vi "Settings.vi"(8 "error in (no error)":errorcluster) -> (0 "error out":errorcluster)   [LabVIEW 2023]
uses:
  <vilib>/Utility/config.llb/Config Data RefNum.ctl
  CTLs/FGV Actions.ctl
  a5ac09e5-38d3-43bc-9feb-68748838b8f7.vi
  <vilib>/Utility/config.llb/Write Key (String).vi
  <vilib>/Utility/config.llb/Read Key (String).vi
  <vilib>/Utility/inputDevices.llb/closeKeyboard.vi
  <vilib>/Utility/inputDevices.llb/keyboardAcquire.vi
  FaKI State Machine/FaKI State Machine.lvlib
  <vilib>/Utility/config.llb/NI_LVConfig.lvlib
panel:
  in  "Reset":bool
  in  "Save":bool
  in  "Current Webhooks":string[][](table)
  in  "Start/Stop":bool
  in  "Exit":bool
  # "Change Hotkey\nPress \"Start Listening\" and hold down a key combination for five seconds to assign it as your new application Hotkey."
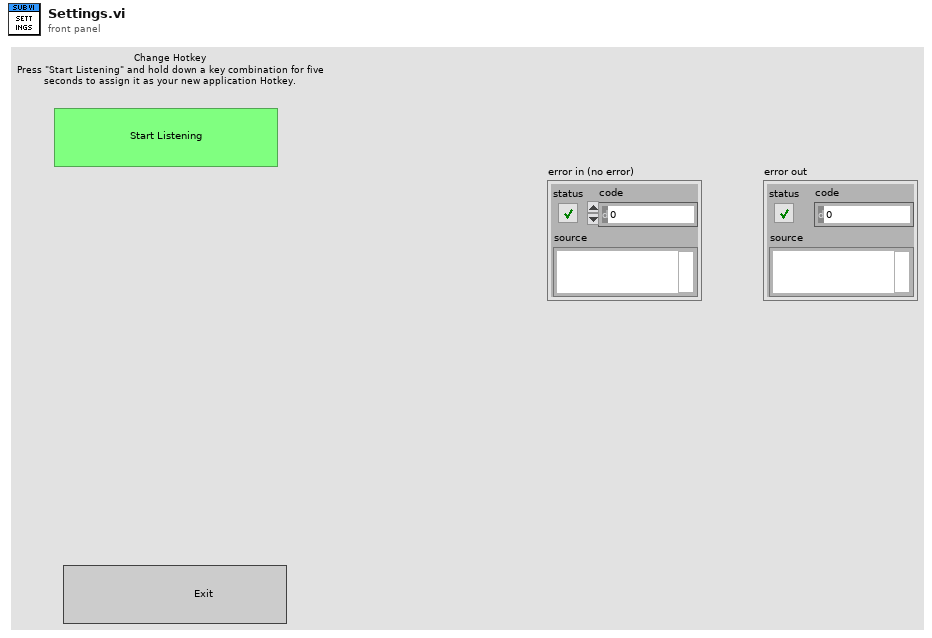
[diagram p1: front panel]
types:
  T1 = enum32{"Invalid", "Standard", "Closed", "Hidden", "Minimized", "Maximized"}
  T2 = enum32{"invalid app kind", "Development System", "Run Time System", "Student Edition", "Embedded LabVIEW", "Evaluation", "Custom"}
  T3 = typedef "FGV Actions.ctl" = enum16{"Read", "Write"}
  T4 = typedef "NI_LVConfig.lvlib/Config Data RefNum.ctl" = refnum<k1>
  T5 = cluster{"Core":cluster{"Current VI Reference":refnum<vi>, "Close Panel on Exit?":bool}, "Config":T4, "Keyboard":refnum<k1>, "Last":enum16{"0", "1", "2", "3", "4", "5", "6", "7", "8", "9", "A", "B", "C", "D", "E", "F", "G", "H", "I", "J", "K", "L", "M", "N", "O", "P", "Q", "R", "S", "T", "U", "V", "W", "X", "Y", "Z", "F1", "F2", "F3", "F4", "F5", "F6", "F7", "F8", "F9", "F10", "F11", "F12", "F13", "F14", "F15", "ADD", "BACK", "BACKSLASH", "CAPITAL", "COMMA", "DECIMAL", "DELETE", "DIVIDE", "DOWN", "END", "EQUALS", "ESCAPE", "GRAVE (`)", "HOME", "INSERT", "LBRACKET", "LCONTROL", "LEFT", "L ALT", "LSHIFT", "LWIN", "MINUS", "MULTIPLY", "NEXT", "NUMLOCK", "NUMPAD_0", "NUMPAD_1", "NUMPAD_2", "NUMPAD_3", "NUMPAD_4", "NUMPAD_5", "NUMPAD_6", "NUMPAD_7", "NUMPAD_8", "NUMPAD_9", "PAUSE", "PERIOD", "PRIOR (PG UP)", "RBRACKET", "RCONTROL", "RETURN", "RIGHT", "R ALT", "RSHIFT", "RWIN", "SCROLL", "SEMICOLON", "SLASH", "SPACE", "SUBTRACT", "TAB", "UP", "ENTER (num pad)", "' (quote)"}[]}
  T6 = enum16{"0", "1", "2", "3", "4", "5", "6", "7", "8", "9", "A", "B", "C", "D", "E", "F", "G", "H", "I", "J", "K", "L", "M", "N", "O", "P", "Q", "R", "S", "T", "U", "V", "W", "X", "Y", "Z", "F1", "F2", "F3", "F4", "F5", "F6", "F7", "F8", "F9", "F10", "F11", "F12", "F13", "F14", "F15", "ADD", "BACK", "BACKSLASH", "CAPITAL", "COMMA", "DECIMAL", "DELETE", "DIVIDE", "DOWN", "END", "EQUALS", "ESCAPE", "GRAVE (`)", "HOME", "INSERT", "LBRACKET", "LCONTROL", "LEFT", "L ALT", "LSHIFT", "LWIN", "MINUS", "MULTIPLY", "NEXT", "NUMLOCK", "NUMPAD_0", "NUMPAD_1", "NUMPAD_2", "NUMPAD_3", "NUMPAD_4", "NUMPAD_5", "NUMPAD_6", "NUMPAD_7", "NUMPAD_8", "NUMPAD_9", "PAUSE", "PERIOD", "PRIOR (PG UP)", "RBRACKET", "RCONTROL", "RETURN", "RIGHT", "R ALT", "RSHIFT", "RWIN", "SCROLL", "SEMICOLON", "SLASH", "SPACE", "SUBTRACT", "TAB", "UP", "ENTER (num pad)", "' (quote)"}[]
  T7 = cluster{"Current VI Reference":refnum<vi>, "Close Panel on Exit?":bool}
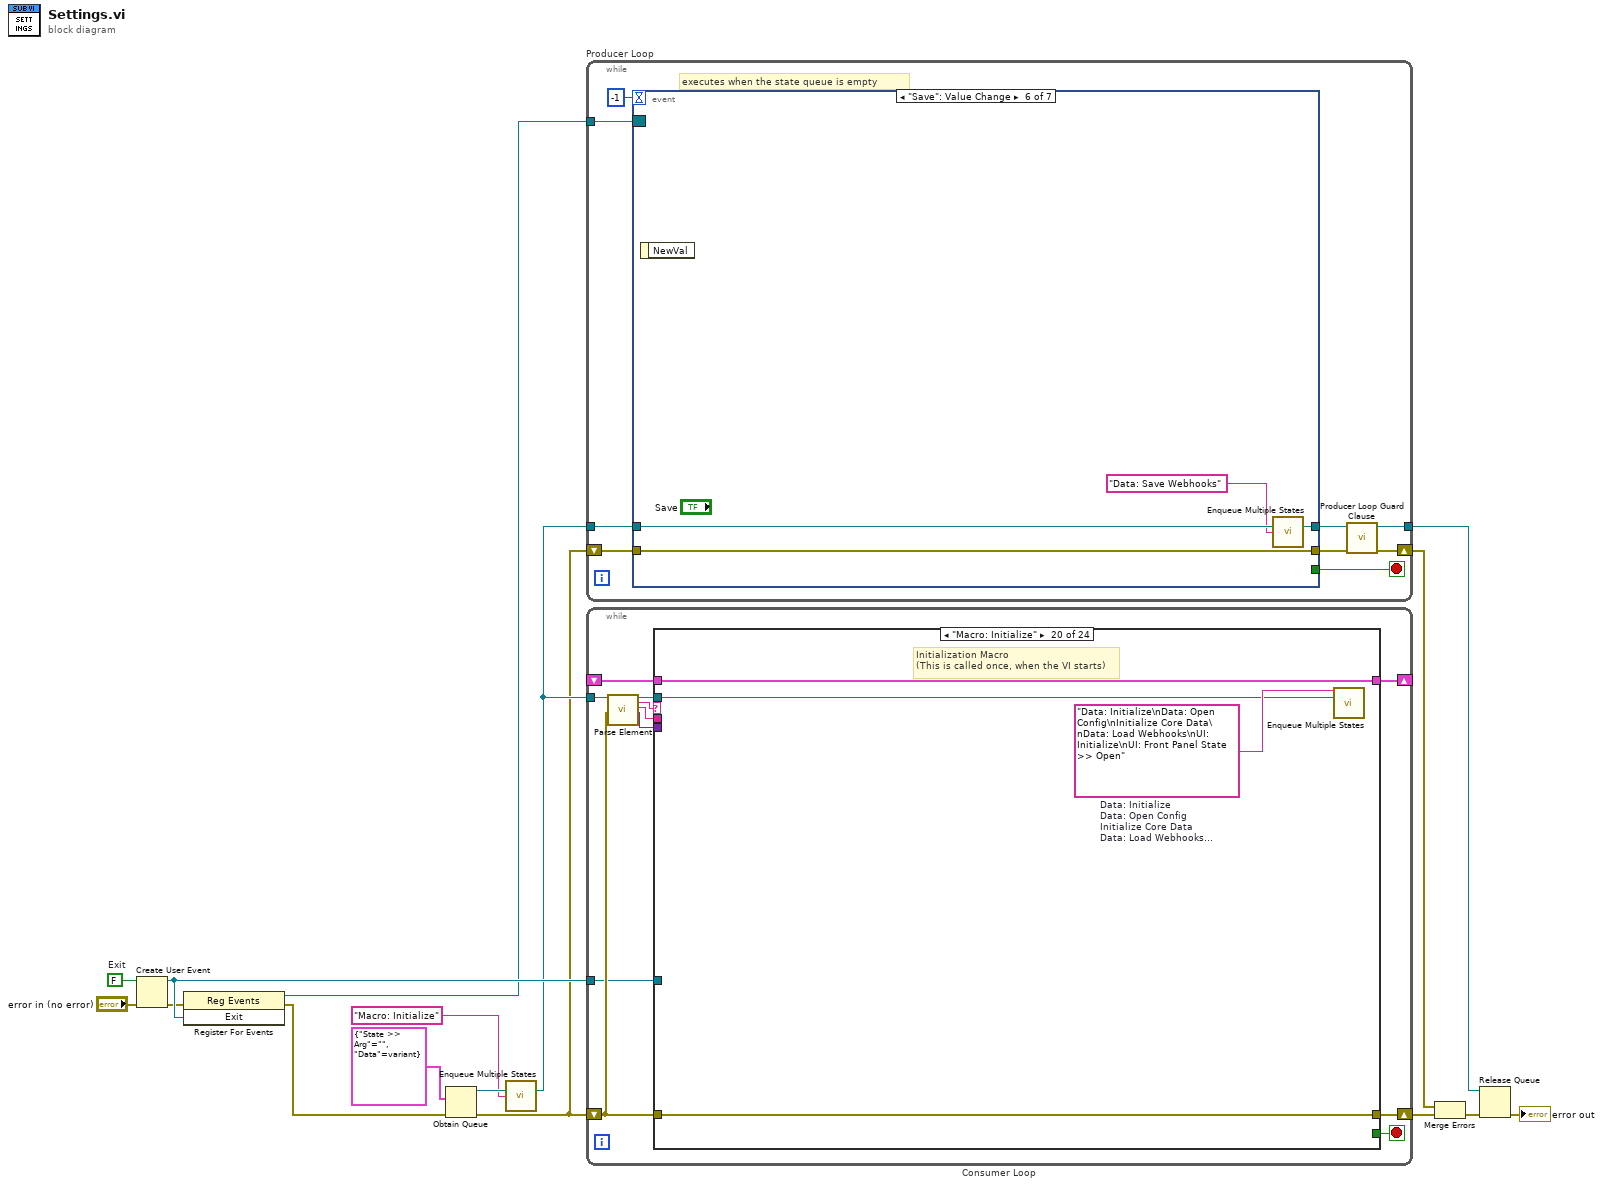
[diagram p0: block diagram]
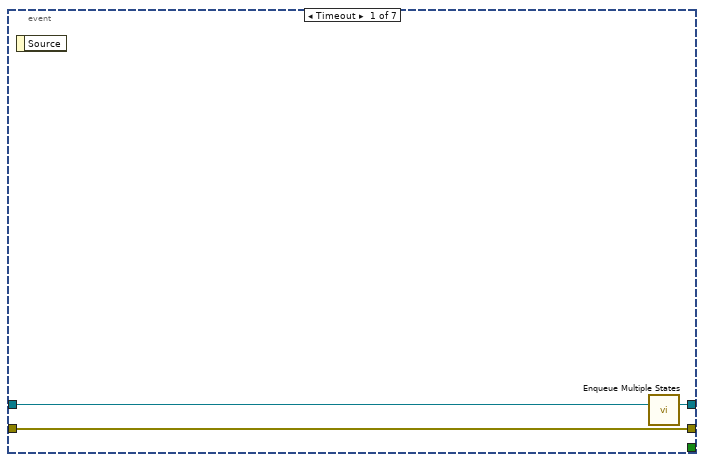
[diagram p2: hidden frame]
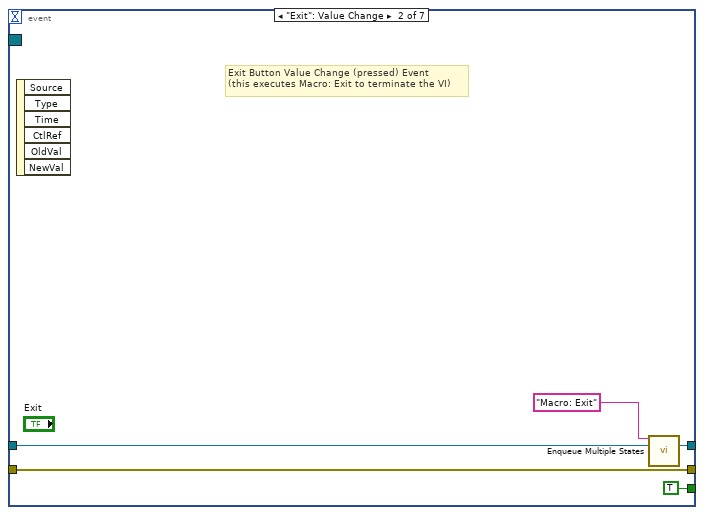
[diagram p3: hidden frame]
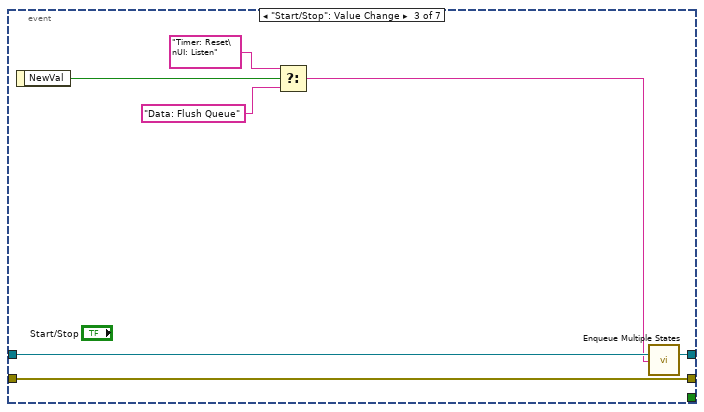
[diagram p4: hidden frame]
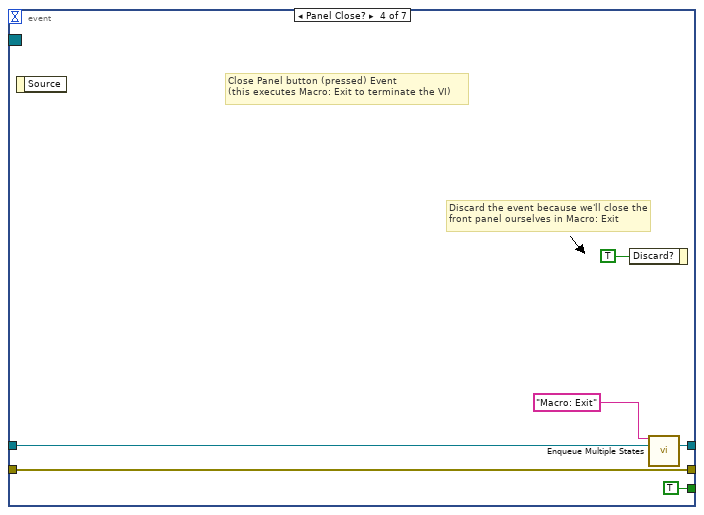
[diagram p5: hidden frame]
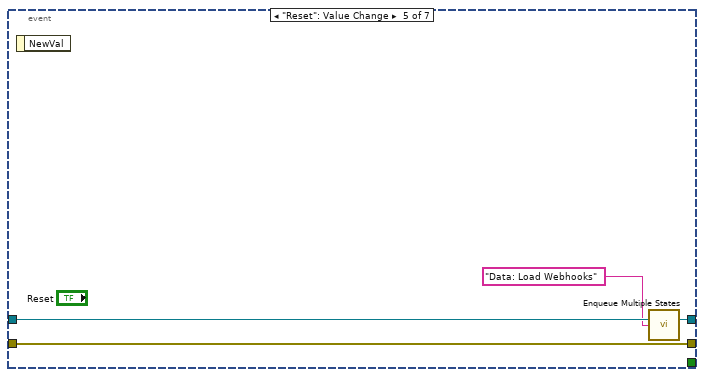
[diagram p6: hidden frame]
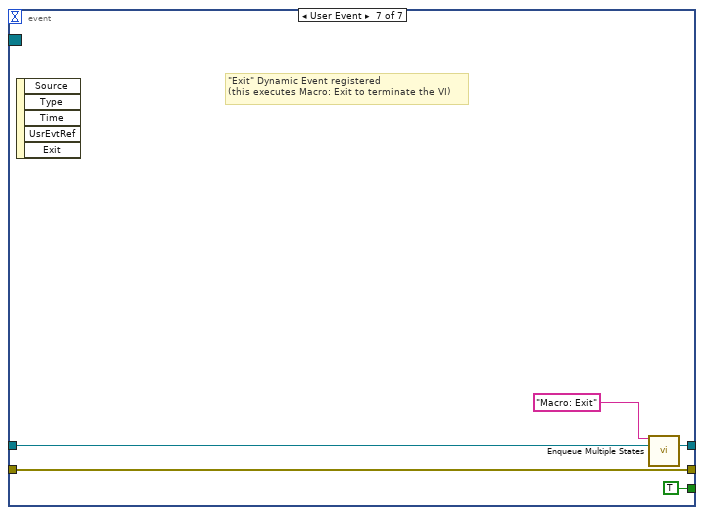
[diagram p7: hidden frame]
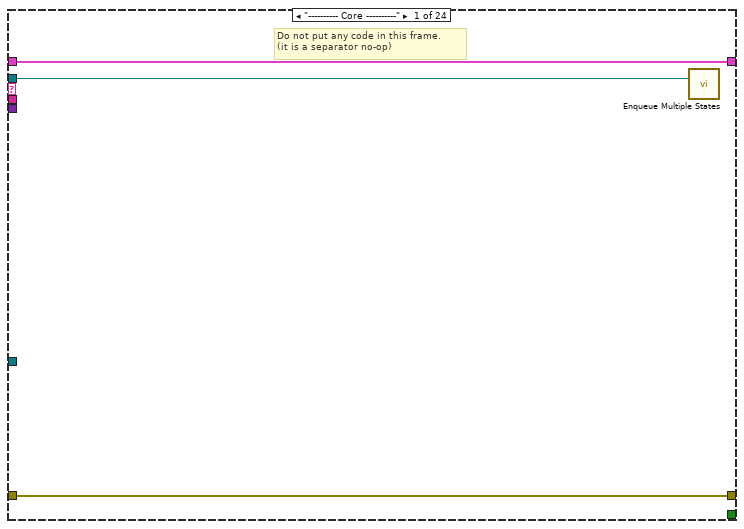
[diagram p8: hidden frame]
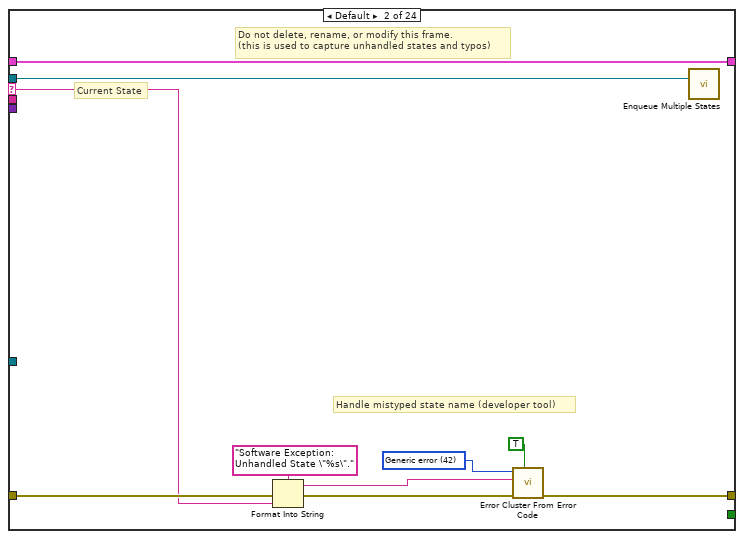
[diagram p9: hidden frame]
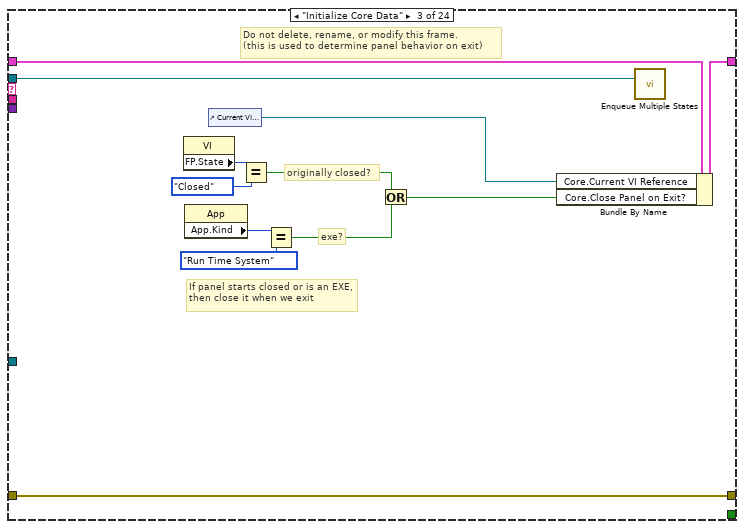
[diagram p10: hidden frame]
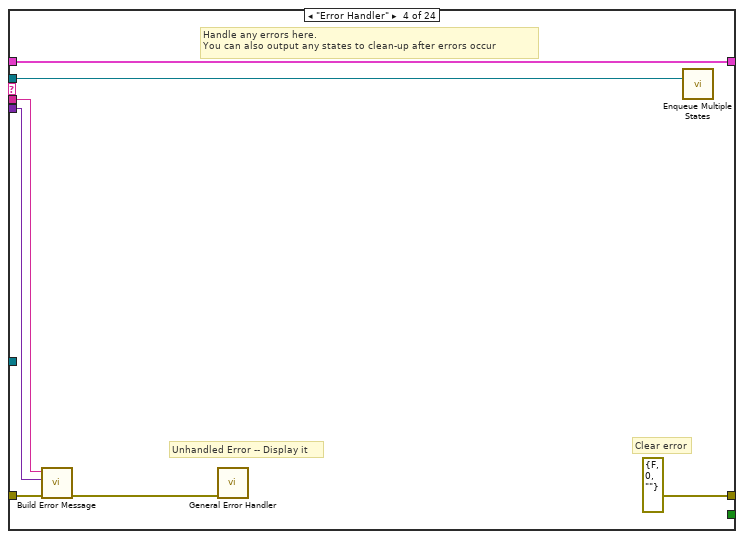
[diagram p11: hidden frame]
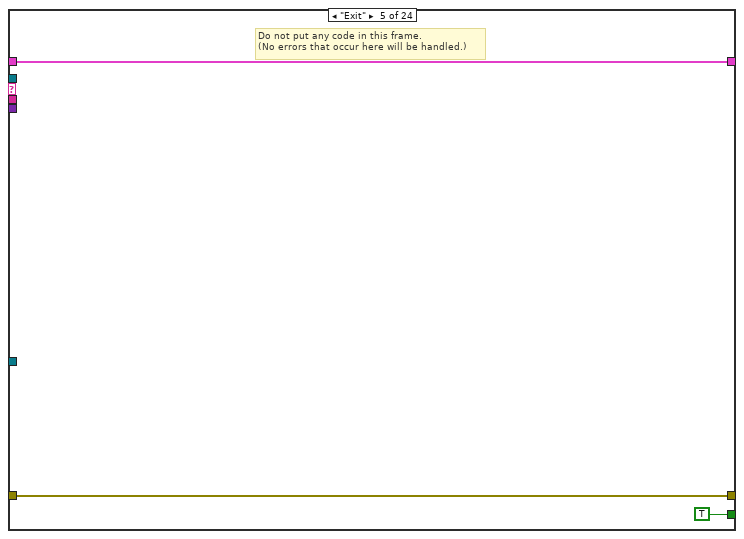
[diagram p12: hidden frame]
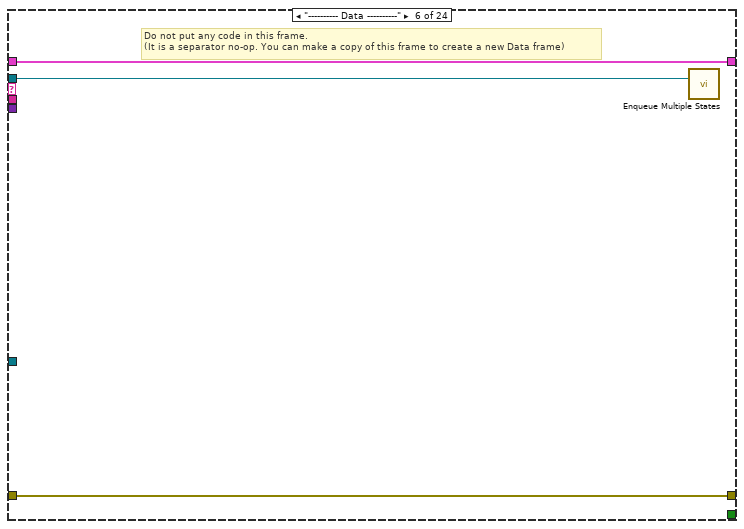
[diagram p13: hidden frame]
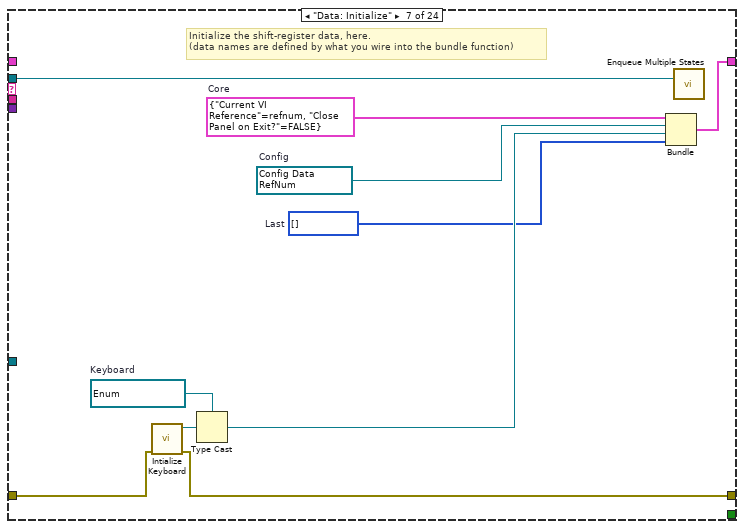
[diagram p14: hidden frame]
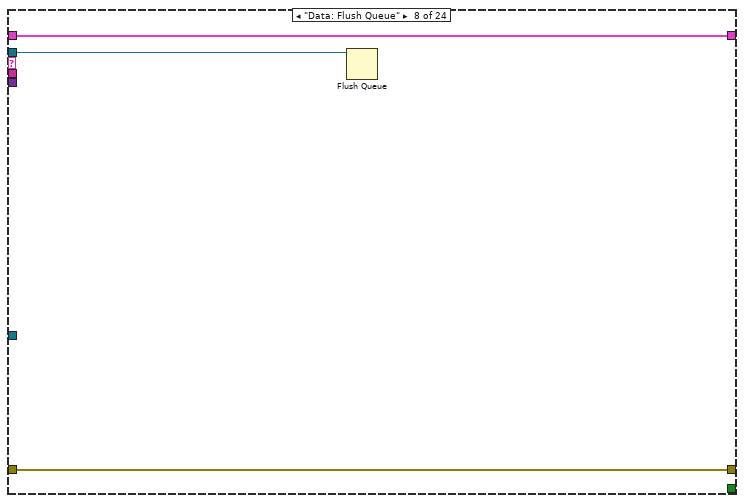
[diagram p15: hidden frame]
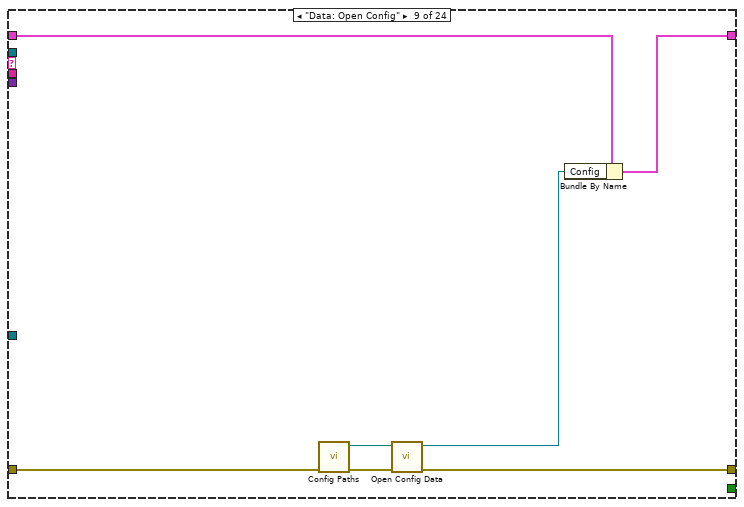
[diagram p16: hidden frame]
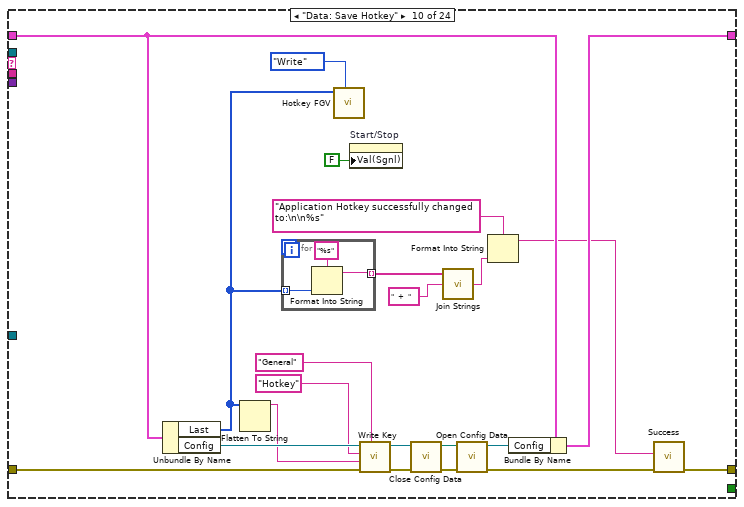
[diagram p17: hidden frame]
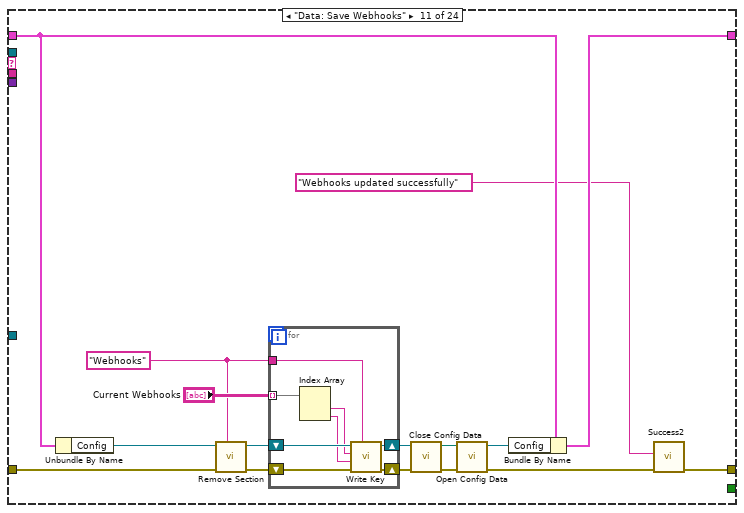
[diagram p18: hidden frame]
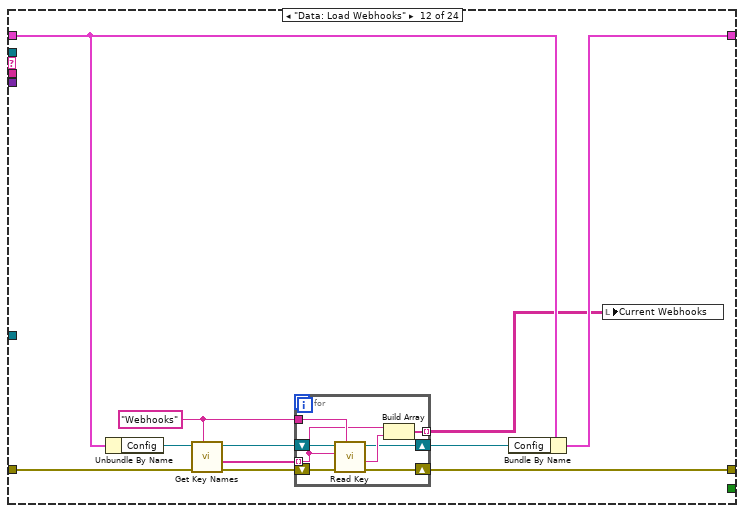
[diagram p19: hidden frame]
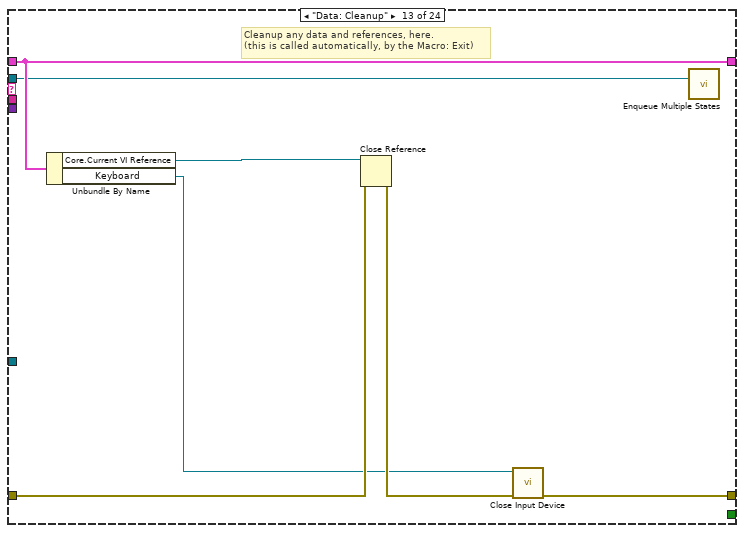
[diagram p20: hidden frame]
diagram:
  w13 = FALSE  # Exit
  n1 = Create User Event(user event datatype=w13, error in="error in (no error)") -> (user event=w16:refnum<user-event>, error out=w12:errorcluster)
  n2 = register-events(error in=w12, w16) -> (reference out=w15:refnum<event-registration>, error out=w14:errorcluster)  [unwired: 1 in]
  n3 = Obtain Queue(element data type=cluster{"State >> Arg":string, "Data":variant} {"State >> Arg"="", "Data"=variant}, error in (no error)=w14) -> (queue out=w6:refnum<queue>, error out=w3:errorcluster)  [unwired: 3 in, 1 out]
  n4 = call "Enqueue Multiple States.vi"("queue in"=w6, "State(s) at Back"="Macro: Initialize") -> ("queue out"=w7:refnum<queue>)  [unwired: 13 in]
  n5 = while "Producer Loop" {
    shift-right: [w20] -> w9
    shift-left: w3 -> [w25]
    tunnel: w15 -> [w17]
    tunnel: w7 -> [w23]
    tunnel: [w18] -> w11
    stop <- w22 stop-if-true
    # "executes when the state queue is empty"
    n6 = event shown="[5] \"Save\": Value Change" {
      selector: w17 -> [_ _ _ _ _ _ _]
      dyn-events: _ -> [_ _ _ _ _ _ _]
      timeout: -1 ("Timeout") -> [_ _ _ _ _ _ _]
      tunnel: [w26 w33 w40 w46 w50 w54 w59] -> w21
      tunnel: w25 -> [w26 w33 w40 w46 w50 w54 w59]
      tunnel: w23 -> [w27 w32 w39 w43 w49 w53 w57]
      tunnel: [w28 w30 w38 w42 w48 w52 w56] -> w19
      tunnel: [_ TRUE _ TRUE _ _ TRUE] -> w22
      event Timeout {
        n7 = event-data() -> ()  [unwired: 1 in, 1 out]
        n8 = call "Enqueue Multiple States.vi"("queue in"=w27) -> ("queue out"=w28:refnum<queue>)  [unwired: 14 in]
      }
      event "Exit": Value Change {
        # "Exit Button Value Change (pressed) Event\n(this executes Macro: Exit to terminate the VI)"
        n9 = event-data() -> ()  [unwired: 1 in, 6 out]
        n10 = call "Enqueue Multiple States.vi"("State(s) at Front"="Macro: Exit", "queue in"=w32) -> ("queue out"=w30:refnum<queue>)  [unwired: 13 in]
      }
      event "Start/Stop": Value Change {
        n11 = event-data() -> ("NewVal"=w37:bool)  [unwired: 1 in]
        n12 = Select(t="Timer: Reset\nUI: Listen", s=w37, f="Data: Flush Queue") -> (s? t:f=w34:string)
        n13 = call "Enqueue Multiple States.vi"("queue in"=w39, "State(s) at Back"=w34) -> ("queue out"=w38:refnum<queue>)  [unwired: 13 in]
      }
      event Panel Close? {
        # "Discard the event because we'll close the front panel ourselves in Macro: Exit"
        # "Close Panel button (pressed) Event\n(this executes Macro: Exit to terminate the VI)"
        n14 = event-data() -> ()  [unwired: 1 in, 1 out]
        n15 = event-data("Discard?"=TRUE) -> ()  [unwired: 1 in, 1 out]
        n16 = call "Enqueue Multiple States.vi"("State(s) at Front"="Macro: Exit", "queue in"=w43) -> ("queue out"=w42:refnum<queue>)  [unwired: 13 in]
      }
      event "Reset": Value Change {
        n17 = event-data() -> ()  [unwired: 1 in, 1 out]
        n18 = call "Enqueue Multiple States.vi"("queue in"=w49, "State(s) at Back"="Data: Load Webhooks") -> ("queue out"=w48:refnum<queue>)  [unwired: 13 in]
      }
      event "Save": Value Change {
        n19 = event-data() -> ()  [unwired: 1 in, 1 out]
        n20 = call "Enqueue Multiple States.vi"("queue in"=w53, "State(s) at Back"="Data: Save Webhooks") -> ("queue out"=w52:refnum<queue>)  [unwired: 13 in]
      }
      event User Event {
        # "\"Exit\" Dynamic Event registered\n(this executes Macro: Exit to terminate the VI)"
        n21 = event-data() -> ()  [unwired: 1 in, 5 out]
        n22 = call "Enqueue Multiple States.vi"("State(s) at Front"="Macro: Exit", "queue in"=w57) -> ("queue out"=w56:refnum<queue>)  [unwired: 13 in]
      }
    }
    n23 = call "Producer Loop Guard Clause.vi"("error in (no error)"=w21, "queue in"=w19) -> ("error out"=w20:errorcluster, "queue out"=w18:refnum<queue>)  [unwired: 8 in]
  }
  n24 = while "Consumer Loop" {
    shift-right: [w67] -> _
    shift-left: _ -> [w66]
    shift-right: [w70] -> w8
    shift-left: w3 -> [w69]
    tunnel: w7 -> [w65]
    tunnel: w16 -> [w60]
    stop <- w68 stop-if-true
    n25 = call "Parse Element.vi"("queue in"=w65, "error in (no error)"=w69) -> ("queue out"=w64:refnum<queue>, "State"=w63:string, "Arg"=w62:string, "Data"=w61:variant)  [unwired: 14 in]
    n26 = case shown="\"Macro: Initialize\"" w63 {
      selector: w63 -> [_ w75 _ _ _ _ _ _ _ _ _ _ _ _ _ _ _ _ _ _ _ _ _ _]
      tunnel: w64 -> [w71 w74 w84 w100 _ w106 w116 w121 _ _ _ _ w200 w204 w207 w210 w219 w294 w308 w311 w318 w324 _ w333]
      tunnel: w62 -> [_ _ _ w96 _ _ _ _ _ _ _ _ _ _ _ w211 w220 _ _ _ _ _ _ _]
      tunnel: w66 -> [w72 w77 w90 w101 w104 w107 _ w120 w125 w149 w168 w187 w201 w205 w208 w212 w222 w293 w309 w313 w322 w325 w331 w340]
      tunnel: [w73 w82 w95 errorcluster {"status"=FALSE, "code"=0, "source"=""} ("error out") w105 w108 w110 w119 w126 w132 w161 w180 w198 w206 w209 w213 w223 w302 w310 w314 w323 w326 w329 w338] -> w70
      tunnel: w69 -> [w73 w81 w95 w99 w105 w108 w113 w119 w127 w148 w158 w186 w203 w206 w209 w214 w224 w303 w310 w314 w323 w326 w330 w339]
      tunnel: [_ _ _ _ TRUE _ _ _ _ _ _ _ _ _ _ _ _ _ _ _ _ _ _ _] -> w68
      tunnel: [w72 w77 w94 w101 w104 w107 w118 w120 w124 w150 w169 w188 w201 w205 w208 w212 w222 w292 w309 w313 w322 w325 w331 w340] -> w67
      tunnel: w61 -> [_ _ _ w97 _ _ _ _ _ _ _ _ _ _ _ _ _ _ _ _ _ _ _ _]
      tunnel: w60 -> [_ _ _ _ _ _ _ _ _ _ _ _ _ _ _ _ _ _ _ _ _ _ _ _]
      frame "---------- Core ----------" {
        # "Do not put any code in this frame.\n(it is a separator no-op)"
        n27 = call "Enqueue Multiple States.vi"("queue in"=w71) -> ()  [unwired: 14 in, 1 out]
      }
      frame Default {
        w79 = 42 items=["No error", "Argument error", "Memory is full", "Out of zone", "End of file", "File already open", "Generic file I/O error", "File not found", "File permission error", "Disk is full", "Duplicate path", "Too many files open", "System feature not enabled", "Resource file not found", "Cannot add resource", "Resource not found", "Image not found", "Image memory error", "Pen does not exist", "Config type invalid", "Config token not found", "Config parse error", "Config memory error", "Bad external code format", "Bad external code offset", "External code not present", "Null window", "Destroy window error", "Null menu", "Print aborted", "Bad print record", "Print driver error", "Windows error during printing", "Memory error during printing", "Print dialog error", "Generic print error", "Invalid device refnum", "Device not found", "Device parameter error", "Device unit error", "Cannot open device", "Device call aborted", "Generic error", "Cancelled by user", "Object ID too low", "Object ID too high", "Object not in heap", "Unknown heap", "Unknown object (invalid DefProc)", "Unknown object (DefProc not in table)", "Message out of range", "Invalid (null) method", "Unknown message", "Manager call not supported", "Bad address", "Network operation in progress", "Network operation timed out", "Connection is busy", "Network attribute not supported", "Network error", "Address in use", "System out of memory", "Connection aborted", "Connection refused", "Not connected", "Already connected", "Connection closed", "Initialization error (interapplication manager)", "Bad occurrence", "Wait on unbound occurrence handler", "Occurrence queue overflow", "Datalog type conflict", "Unused", "Unrecognized type (interapplication manager)", "Memory corrupt", "Failed to make temporary DLL", "Old CIN version", "Drag socket not found", "Failed to load drop-object", "Failed to register OLE object", "Failed to release OLE object", "Format specifier type mismatch", "Unknown format specifier", "Too few format specifiers", "Too many format specifiers", "Scan failed", "Newer CIN version", "Error converting to variant", "Runtime menu error", "Password tampered", "Variant attribute not found", "Incompatible variant data type", "Event data is not available", "Event Store is not present", "Occurrence is not found", "Event Queue is not created", "Event info is not available", "Refnum passed is NULL", "Error retrieving Class GUID", "Error retrieving CoClass GUID", "Error retrieving TypeLib GUID.", "Bad built application magic bytes.", "Specific driver is different from the specific driver associated with the Logical Name.", "There is no session opened to the class driver.", "Max Error", "MAX - Error with config objects", "MAX - Error loading configuration", "MAX - Group not supported"]
        # "Current State"
        # "Do not delete, rename, or modify this frame.\n(this is used to capture unhandled states and typos)"
        # "Handle mistyped state name (developer tool)"
        n28 = Format Into String(format string="Software Exception: Unhandled State \"%s\"." ("message"), error in=w81, w75) -> (resulting string=w78:string, error out=w83:errorcluster)  [unwired: 1 in]
        n29 = call <vilib>:"Error Cluster From Error Code.vi"("show call chain? (False)"=TRUE, "error in (no error)"=w83, "error message (\"\")"=w78, "error code (0)"=w79) -> ("error out"=w82:errorcluster)  [unwired: 5 in]
        n30 = call "Enqueue Multiple States.vi"("queue in"=w74) -> ()  [unwired: 14 in, 1 out]
      }
      frame "Initialize Core Data" {
        # "Do not delete, rename, or modify this frame.\n(this is used to determine panel behavior on exit)"
        # "originally closed?"
        # "exe?"
        # "If panel starts closed or is an EXE, then close it when we exit"
        n31 = property class="VI"() -> ("FP.State"=w87:T1)  [unwired: 2 in, 2 out]
        n32 = property class="App"() -> ("App.Kind"=w93:T2)  [unwired: 2 in, 2 out]
        n33 = control-ref of="Current VI Reference"() -> (w88:refnum<vi>)
        n34 = Equal?(x=w87, y=T1."Closed" ("Front Panel Window:State")) -> (x = y?=w85:bool)
        n35 = Equal?(x=w93, y=T2."Run Time System" ("Application:Kind")) -> (x = y?=w91:bool)
        n36 = Or(x=w85, y=w91) -> (x .or. y?=w89:bool)
        n37 = Bundle By Name(cluster=w90, "Core.Current VI Reference"=w88, "Core.Close Panel on Exit?"=w89) -> (w94:T5)
        n38 = call "Enqueue Multiple States.vi"("queue in"=w84) -> ()  [unwired: 14 in, 1 out]
      }
      frame "Error Handler" {
        # "Unhandled Error -- Display it"
        # "Handle any errors here.\nYou can also output any states to clean-up after errors occur"
        # "Clear error"
        n39 = call "Build Error Message.vi"("error in (no error)"=w99, "Data"=w97, "Arg"=w96) -> ("error out"=w98:errorcluster)  [unwired: 8 in]
        n40 = call <vilib>:"General Error Handler.vi"("error in (no error)"=w98) -> ()  [unwired: 10 in, 5 out]
        n41 = call "Enqueue Multiple States.vi"("queue in"=w100) -> ()  [unwired: 14 in, 1 out]
      }
      frame "Exit" {
        # "Do not put any code in this frame.\n(No errors that occur here will be handled.)"
      }
      frame "---------- Data ----------" {
        # "Do not put any code in this frame.\n(It is a separator no-op. You can make a copy of this frame to create a new Data frame)"
        n42 = call "Enqueue Multiple States.vi"("queue in"=w106) -> ()  [unwired: 14 in, 1 out]
      }
      frame "Data: Initialize" {
        w109 = T6 [] items=["0", "1", "2", "3", "4", "5", "6", "7", "8", "9", "A", "B", "C", "D", "E", "F", "G", "H", "I", "J", "K", "L", "M", "N", "O", "P", "Q", "R", "S", "T", "U", "V", "W", "X", "Y", "Z", "F1", "F2", "F3", "F4", "F5", "F6", "F7", "F8", "F9", "F10", "F11", "F12", "F13", "F14", "F15", "ADD", "BACK", "BACKSLASH", "CAPITAL", "COMMA", "DECIMAL", "DELETE", "DIVIDE", "DOWN", "END", "EQUALS", "ESCAPE", "GRAVE (`)", "HOME", "INSERT", "LBRACKET", "LCONTROL", "LEFT", "L ALT", "LSHIFT", "LWIN", "MINUS", "MULTIPLY", "NEXT", "NUMLOCK", "NUMPAD_0", "NUMPAD_1", "NUMPAD_2", "NUMPAD_3", "NUMPAD_4", "NUMPAD_5", "NUMPAD_6", "NUMPAD_7", "NUMPAD_8", "NUMPAD_9", "PAUSE", "PERIOD", "PRIOR (PG UP)", "RBRACKET", "RCONTROL", "RETURN", "RIGHT", "R ALT", "RSHIFT", "RWIN", "SCROLL", "SEMICOLON", "SLASH", "SPACE", "SUBTRACT", "TAB", "UP", "ENTER (num pad)", "' (quote)"]  # Last
        w112 = T4 refnum items=["config data"]  # Config
        w114 = refnum<k1> refnum items=["KEYBOARD"]  # Keyboard
        w117 = T7 {"Current VI Reference"=refnum, "Close Panel on Exit?"=FALSE}  # Core
        # "Initialize the shift-register data, here.\n(data names are defined by what you wire into the bundle function)"
        n43 = call <vilib>:"Intialize Keyboard.vi"("error in (no error)"=w113) -> ("error out"=w110:errorcluster, "device ID"=w115:refnum<k1>)  [unwired: 9 in]
        n44 = Type Cast(type=w114, x=w115) -> (*(type *) &x=w111:refnum<k1>)
        n45 = Bundle("Core"=w117, "Config"=w112, "Keyboard"=w111, "Last"=w109) -> (w118:T5)  [unwired: 1 in]
        n46 = call "Enqueue Multiple States.vi"("queue in"=w116) -> ()  [unwired: 14 in, 1 out]
      }
      frame "Data: Flush Queue" {
        n47 = Flush Queue(queue=w121) -> ()  [unwired: 1 in, 3 out]
      }
      frame "Data: Open Config" {
        n48 = call "Config Paths.vi"("error in (no error)"=w127) -> ("error out"=w128:errorcluster, "Global Config"=w122:path)  [unwired: 7 in, 2 out]
        n49 = call <vilib>:"Open Config Data.vi"("error in (no error)"=w128, "configuration file path"=w122) -> ("error out"=w126:errorcluster, "refnum"=w123:T4)  [unwired: 7 in, 1 out]
        n50 = Bundle By Name(cluster=w125, "Config"=w123) -> (w124:T5)
      }
      frame "Data: Save Hotkey" {
        n51 = Unbundle By Name(w149) -> ("Last"=w130:T6, "Config"=w143:T4)
        n52 = Flatten To String(anything=w130) -> (data string=w142:string)  [unwired: 3 in, 2 out]
        n53 = for {
          tunnel: w130 -> [w152] mode=indexing
          tunnel: [w151] -> w138 mode=indexing
          n54 = Format Into String(format string="%s", w152) -> (resulting string=w151:string)  [unwired: 2 in, 1 out]
        }
        n55 = call "Hotkey FGV.vi"("Mode"=FGV_Actions."Write", "Hotkey"=w130) -> ()  [unwired: 7 in, 3 out]
        n56 = property on="Start/Stop" class="Bool (strict)"("Val(Sgnl)"=FALSE ("Value (Signaling)")) -> ()  [unwired: 2 in, 2 out]
        n57 = call-poly <vilib>:"Write Key.vi"("section"="General", "error in (no error)"=w148, "value"=w142, "key"="Hotkey", "refnum"=w143) -> ("error out"=w147:errorcluster, "refnum out"=w146:T4)  [unwired: 4 in, 1 out]
        n58 = call <vilib>:"Close Config Data.vi"("error in (no error)"=w147, "refnum"=w146) -> ("error out"=w144:errorcluster, "file path"=w145:path)  [unwired: 8 in]
        n59 = call <vilib>:"Join Strings.vi"("Separator (,)"="  +  ", "Strings In"=w138) -> ("String"=w135:string)  [unwired: 1 in]
        n60 = call <vilib>:"Open Config Data.vi"("error in (no error)"=w144, "configuration file path"=w145) -> ("error out"=w133:errorcluster, "refnum"=w139:T4)  [unwired: 7 in, 1 out]
        n61 = Format Into String(format string="Application Hotkey successfully changed to:\n\n%s", w135) -> (resulting string=w134:string)  [unwired: 2 in, 1 out]
        n62 = Bundle By Name(cluster=w149, "Config"=w139) -> (w150:T5)
        n63 = call "Success"("error in (no error)"=w133, "Message"=w134) -> ("error out"=w132:errorcluster)  [unwired: 8 in, 1 out]
      }
      frame "Data: Save Webhooks" {
        w155 = "Webhooks" ("section")
        n64 = Unbundle By Name(w168) -> ("Config"=w156:T4)
        n65 = call <vilib>:"Remove Section.vi"("section"=w155, "error in (no error)"=w158, "refnum"=w156) -> ("error out"=w154:errorcluster, "refnum out"=w157:T4)  [unwired: 6 in, 1 out]
        n66 = for {
          tunnel: w155 -> [w173]
          shift-right: [w176] -> w167
          shift-left: w154 -> [w177]
          tunnel: "Current Webhooks" -> [w172] mode=indexing
          shift-right: [w175] -> w166
          shift-left: w157 -> [w174]
          n67 = Index Array(array=w172) -> (element #1=w170:string, element #2=w171:string)  [unwired: 2 in]
          n68 = call-poly <vilib>:"Write Key.vi"("section"=w173, "error in (no error)"=w177, "value"=w171, "key"=w170, "refnum"=w174) -> ("error out"=w176:errorcluster, "refnum out"=w175:T4)  [unwired: 4 in, 1 out]
        }
        n69 = call <vilib>:"Close Config Data.vi"("error in (no error)"=w167, "refnum"=w166) -> ("error out"=w164:errorcluster, "file path"=w165:path)  [unwired: 8 in]
        n70 = call <vilib>:"Open Config Data.vi"("error in (no error)"=w164, "configuration file path"=w165) -> ("error out"=w162:errorcluster, "refnum"=w163:T4)  [unwired: 7 in, 1 out]
        n71 = Bundle By Name(cluster=w168, "Config"=w163) -> (w169:T5)
        n72 = call "Success2"("error in (no error)"=w162, "Message"="Webhooks updated successfully") -> ("error out"=w161:errorcluster)  [unwired: 8 in, 1 out]
      }
      frame "Data: Load Webhooks" {
        w181 = "Webhooks" ("section")
        n73 = Unbundle By Name(w187) -> ("Config"=w185:T4)
        n74 = call <vilib>:"Get Key Names.vi"("section"=w181, "error in (no error)"=w186, "refnum"=w185) -> ("error out"=w183:errorcluster, "key names"=w182:string[], "refnum out"=w184:T4)  [unwired: 5 in, 1 out]
        n75 = for {
          tunnel: w182 -> [w193] mode=indexing
          tunnel: w181 -> [w194]
          tunnel: [w191] -> w178 mode=indexing
          shift-right: [w190] -> w180
          shift-left: w183 -> [w195]
          shift-right: [w189] -> w179
          shift-left: w184 -> [w196]
          n76 = call-poly <vilib>:"Read Key.vi"("section"=w194, "error in (no error)"=w195, "key"=w193, "refnum"=w196) -> ("error out"=w190:errorcluster, "value"=w192:string, "refnum out"=w189:T4)  [unwired: 4 in, 1 out]
          n77 = Build Array(w193, w192) -> (w191:string[])
        }
        n78 = Bundle By Name(cluster=w187, "Config"=w179) -> (w188:T5)
        n79 = local write "Current Webhooks"(w178) -> ()
      }
      frame "Data: Cleanup" {
        # "Cleanup any data and references, here.\n(this is called automatically, by the Macro: Exit)"
        n80 = Unbundle By Name(w201) -> ("Core.Current VI Reference"=w202:refnum<vi>, "Keyboard"=w197:refnum<k1>)
        n81 = Close Reference(reference=w202, error in (no error)=w203) -> (error out=w199:errorcluster)
        n82 = call-poly <vilib>:"Close Input Device.vi"("error in (no error)"=w199, "device ID"=w197) -> ("error out"=w198:errorcluster)  [unwired: 8 in]
        n83 = call "Enqueue Multiple States.vi"("queue in"=w200) -> ()  [unwired: 14 in, 1 out]
      }
      frame "---------- UI ----------" {
        # "Do not put any code in this frame.\n(It is a separator no-op. You can make a copy of this frame to create a new UI frame)"
        n84 = call "Enqueue Multiple States.vi"("queue in"=w204) -> ()  [unwired: 14 in, 1 out]
      }
      frame "UI: Initialize" {
        # "Initialize the User Interface, here.\n(this is called automatically, by the Macro: Init)"
        n85 = call "Enqueue Multiple States.vi"("queue in"=w207) -> ()  [unwired: 14 in, 1 out]
      }
      frame "UI: Cursor Set" {
        # "Argument"
        # "Set and Unset Cursor Busy.\n(Usage: \"UI: Cursor Set >> Busy|Idle\")"
        n86 = case shown="\"Idle\", Default" w211 {
          tunnel: w214 -> [w216 w218]
          tunnel: [w215 w217] -> w213
          frame "Idle", Default {
            n87 = call <vilib>:"Unset Busy.vi"("error in (no error)"=w216) -> ("error out"=w215:errorcluster)  [unwired: 10 in]
          }
          frame "Busy" {
            n88 = call <vilib>:"Set Busy.vi"("error in (no error)"=w218) -> ("error out"=w217:errorcluster)  [unwired: 9 in, 1 out]
          }
        }
        n89 = call "Enqueue Multiple States.vi"("queue in"=w210) -> ()  [unwired: 14 in, 1 out]
      }
      frame "UI: Front Panel State" {
        # "Argument"
        # "Set Front Panel Open or Closed\n(Usage: \"UI: Front Panel State >> Open|Close\")"
        n90 = Unbundle By Name(w222) -> ("Core.Current VI Reference"=w221:refnum<vi>)
        n91 = case shown="\"Open\", \"Standard\", Default" w220 {
          tunnel: w224 -> [w231 w245 w257 w270 w283]
          tunnel: [w232 w246 w258 w271 w284] -> w223
          tunnel: w221 -> [w229 w243 w255 w268 w281]
          frame "Open", "Standard", Default {
            w225 = T1."Standard" ("State")
            n92 = property class="VI"(reference=w229, error in=w231) -> (reference out=w228:refnum<vi>, error out=w230:errorcluster, "FP.State"=w227:T1)
            n93 = Not Equal?(x=w227, y=w225) -> (x != y?=w226:bool)
            n94 = case shown="True" w226 {
              tunnel: [w237 w238] -> w232
              tunnel: w230 -> [w236 w238]
              tunnel: w228 -> [w234 _]
              tunnel: w225 -> [w233 _]
              frame True {
                n95 = invoke class="VI" method="FP.Open"(reference=w234, error in=w236, "Activate"=TRUE, "State"=w233) -> (error out=w237:errorcluster)  [unwired: 1 in, 4 out]
              }
              frame False {
              }
            }
          }
          frame "Close", "Closed" {
            n96 = property class="VI"(reference=w243, error in=w245) -> (reference out=w242:refnum<vi>, error out=w244:errorcluster, "FP.State"=w240:T1)
            n97 = Not Equal?(x=w240, y=T1."Closed" ("Front Panel Window:State")) -> (x != y?=w239:bool)
            n98 = case shown="True" w239 {
              tunnel: [w247 w250] -> w246
              tunnel: w244 -> [w247 w249]
              tunnel: w242 -> [_ w248]
              frame False {
              }
              frame True {
                n99 = invoke class="VI" method="FP.Close"(reference=w248, error in=w249) -> (error out=w250:errorcluster)  [unwired: 1 in, 2 out]
              }
            }
          }
          frame "Hidden", "Hide" {
            w251 = T1."Hidden" ("State")
            n100 = property class="VI"(reference=w255, error in=w257) -> (reference out=w254:refnum<vi>, error out=w256:errorcluster, "FP.State"=w253:T1)
            n101 = Not Equal?(x=w253, y=w251) -> (x != y?=w252:bool)
            n102 = case shown="True" w252 {
              tunnel: [w262 w263] -> w258
              tunnel: w256 -> [w261 w263]
              tunnel: w254 -> [w260 _]
              tunnel: w251 -> [w259 _]
              frame True {
                n103 = invoke class="VI" method="FP.Open"(reference=w260, error in=w261, "State"=w259) -> (error out=w262:errorcluster)  [unwired: 2 in, 4 out]
              }
              frame False {
              }
            }
          }
          frame "Minimize", "Minimized" {
            w264 = T1."Minimized" ("State")
            n104 = property class="VI"(reference=w268, error in=w270) -> (reference out=w267:refnum<vi>, error out=w269:errorcluster, "FP.State"=w266:T1)
            n105 = Not Equal?(x=w266, y=w264) -> (x != y?=w265:bool)
            n106 = case shown="True" w265 {
              tunnel: [w275 w276] -> w271
              tunnel: w269 -> [w274 w276]
              tunnel: w267 -> [w273 _]
              tunnel: w264 -> [w272 _]
              frame True {
                n107 = invoke class="VI" method="FP.Open"(reference=w273, error in=w274, "State"=w272) -> (error out=w275:errorcluster)  [unwired: 2 in, 4 out]
              }
              frame False {
              }
            }
          }
          frame "Maximize", "Maximized" {
            w277 = T1."Maximized" ("State")
            n108 = property class="VI"(reference=w281, error in=w283) -> (reference out=w280:refnum<vi>, error out=w282:errorcluster, "FP.State"=w279:T1)
            n109 = Not Equal?(x=w279, y=w277) -> (x != y?=w278:bool)
            n110 = case shown="True" w278 {
              tunnel: [w288 w289] -> w284
              tunnel: w282 -> [w287 w289]
              tunnel: w280 -> [w286 _]
              tunnel: w277 -> [w285 _]
              frame True {
                n111 = invoke class="VI" method="FP.Open"(reference=w286, error in=w287, "State"=w285) -> (error out=w288:errorcluster)  [unwired: 2 in, 4 out]
              }
              frame False {
              }
            }
          }
        }
        n112 = call "Enqueue Multiple States.vi"("queue in"=w219) -> ()  [unwired: 14 in, 1 out]
      }
      frame "UI: Listen" {
        n113 = Unbundle By Name(w293) -> ("Last"=w300:T6, "Keyboard"=w307:refnum<k1>)
        n114 = call "Stall Data Flow.vim"("value in"=w307, "milliseconds to wait"=u32 1) -> ("value out"=w305:refnum<k1>)  [unwired: 1 out]
        n115 = call-poly <vilib>:"Acquire Input Data.vi"("device ID"=w305, "error in (no error)"=w303) -> ("keys pressed"=w306:T6, "error out"=w302:errorcluster)  [unwired: 15 in, 1 out]
        n116 = Empty Array?(array=w300) -> (empty?=w301:bool)
        n117 = Sort 1D Array(array=w306) -> (sorted array=w291:T6)
        n118 = Not(x=w301) -> (.not. x?=w298:bool)
        n119 = Equal?(x=w300, y=w291) -> (x = y?=w299:bool)
        n120 = And(x=w298, y=w299) -> (x .and. y?=w297:bool)
        n121 = Select(t="Timer: Poll", s=w297, f="Timer: Reset\nUI: Listen") -> (s? t:f=w290:string)
        n122 = call "Enqueue Multiple States.vi"("queue in"=w294, "State(s) at Back"=w290) -> ()  [unwired: 13 in, 1 out]
        n123 = Bundle By Name(cluster=w293, "Last"=w291) -> (w292:T5)
      }
      frame "---------- Macro ----------" {
        # "Do not put any code in this frame.\n(It is a separator no-op. You can make a copy of this frame to create a new Macro frame)"
        n124 = call "Enqueue Multiple States.vi"("queue in"=w308) -> ()  [unwired: 14 in, 1 out]
      }
      frame "Macro: Initialize" {
        w312 = "Data: Initialize\nData: Open Config\nInitialize Core Data\nData: Load Webhooks\nUI: Initialize\nUI: Front Panel State >> Open"  # Data: Initialize Data: Open Config Initialize Core Data Data: Load Webhooks UI: Initialize UI: Front Panel State >> Open
        # "Initialization Macro\n(This is called once, when the VI starts)"
        n125 = call "Enqueue Multiple States.vi"("State(s) at Front"=w312, "queue in"=w311) -> ()  [unwired: 13 in, 1 out]
      }
      frame "Macro: Exit" {
        # "Exit Macro\n(This is called once, when the VI exits)"
        n126 = Unbundle By Name(w322) -> ("Core.Close Panel on Exit?"=w321:bool)
        n127 = Select(t="UI: Front Panel State >> Close\n", s=w321, f="") -> (s? t:f=w317:string)
        n128 = Concatenate Strings(w317, "Data: Cleanup\nExit") -> (w315:string)
        n129 = call "Enqueue Multiple States.vi"("State(s) at Front"=w315, "queue in"=w318) -> ()  [unwired: 13 in, 1 out]
      }
      frame "---------- Timer ----------" {
        # "Template Separator\n(You can make a copy of, or modify, this frame)"
        n130 = call "Enqueue Multiple States.vi"("queue in"=w324) -> ()  [unwired: 14 in, 1 out]
      }
      frame "Timer: Reset" {
        n131 = call "Timer FGV.vi"("Mode"=FGV_Actions."Write", "error in (no error)"=w330, "Timer Value (s)"=5.0) -> ("error out"=w329:errorcluster)  [unwired: 6 in, 2 out]
      }
      frame "Timer: Poll" {
        n132 = call "Timer FGV.vi"("Mode"=FGV_Actions."Read", "error in (no error)"=w339) -> ("error out"=w338:errorcluster, "Expired?"=w336:bool)  [unwired: 7 in, 1 out]
        n133 = Select(t="Data: Save Hotkey", s=w336, f="UI: Listen") -> (s? t:f=w332:string)
        n134 = call "Enqueue Multiple States.vi"("queue in"=w333, "State(s) at Back"=w332) -> ()  [unwired: 13 in, 1 out]
      }
    }
  }
  n135 = Merge Errors(w9, w8) -> (w10:errorcluster)
  n136 = Release Queue(queue=w11, error in (no error)=w10) -> (error out=→"error out":errorcluster)  [unwired: 1 in, 2 out]
